vi "initialise.vi"(8 "error in (no error)":errorcluster, 11 "DL090215DataCollection in":refnum<class "DataCollectionMG091001IntrinsicImaging.lvclass">) -> (0 "error out":errorcluster, 3 "DL090215DataCollection out":refnum<class "DataCollectionMG091001IntrinsicImaging.lvclass">)   [LabVIEW 2010, in "DataCollectionMG091001IntrinsicImaging.lvclass"]
uses:
  DataCollectionMG091001IntrinsicImaging.lvclass
  common/enumerations/top-level_component_type_enum.ctl
  DataCollectionDL091104Scaffold/DataCollectionDL091104Scaffold/DataCollectionDL091104Scaffold.lvclass
  common/classes/ImageCollection/ImageCollection/storage_mode_enum.ctl
  DataCollectionMG091001IntrinsicImaging.lvclass/DataCollectionMG091001IntrinsicImaging.ctl
  common/classes/ImageCollection/ImageCollection/ImageCollection.lvclass
  common/classes/ErrorController/ErrorController/class_data.vi
  common/classes/ErrorController/ErrorController/ErrorController.lvclass
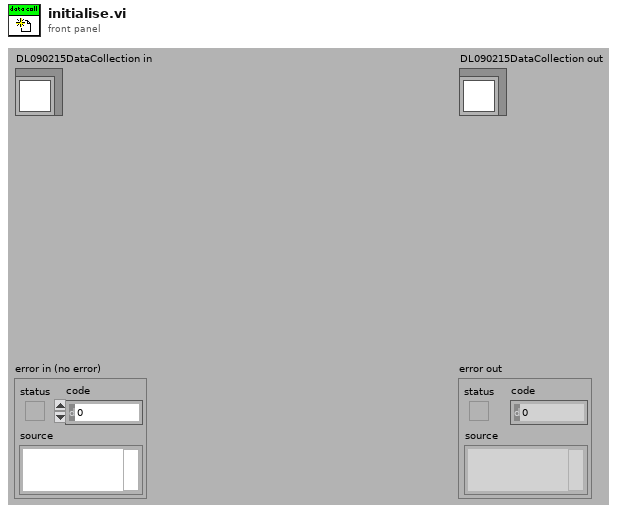
[diagram p1: front panel]
types:
  T1 = typedef "top-level_component_type_enum.ctl" = enum16{"undefined", "ImagingMode", "ScanHead", "DAQ", "ImageAssembler", "Display", "DataCollection", "Analyser", "Stimulator", "ExperimentController", "Instrument", "Stage"}
  T2 = typedef "ImageCollection.lvclass/storage_mode_enum.ctl" = enum16{"RAM", "single files", "multipage TIFF (read-only)"}
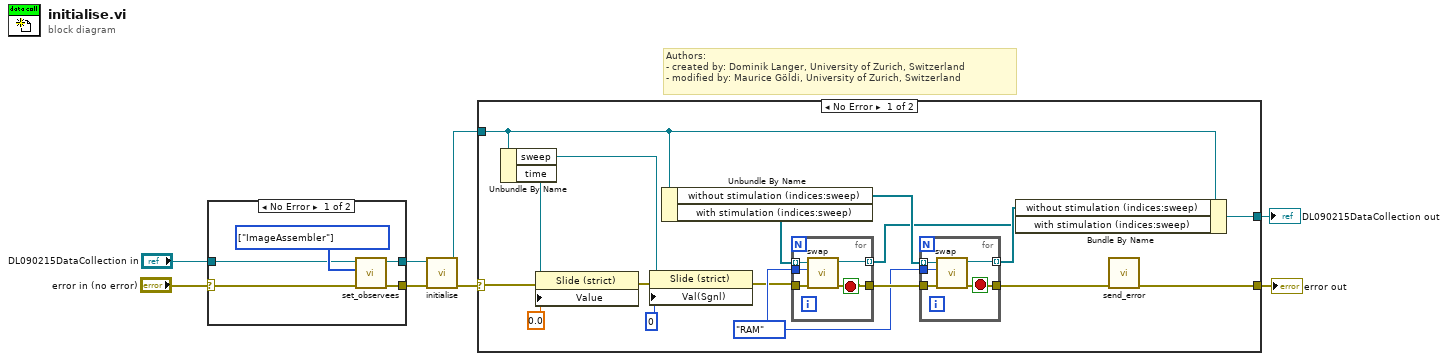
[diagram p0: block diagram]
diagram:
  # "Authors: \n- created by: Dominik Langer, University of Zurich, Switzerland\n- modified by: Maurice Göldi, University of Zurich, Switzerland"
  n1 = case shown="No Error" "error in (no error)" {
    selector: "error in (no error)" -> [w9 w15]
    tunnel: [w12 w15] -> w4
    tunnel: [w11 w14] -> w3
    tunnel: "DL090215DataCollection in" -> [w10 w14]
    frame No Error {
      w13 = T1[] [enum."ImageAssembler"] items=["undefined", "ImagingMode", "ScanHead", "DAQ", "ImageAssembler", "Display", "DataCollection", "Analyser", "Stimulator", "ExperimentController", "Instrument", "Stage"] ("observees")
      n2 = call-dynamic "set_observees.vi"("error in (no error)"=w9, "observees"=w13, "GenericToplevelComponent in"=w10) -> ("error out"=w12:errorcluster, "GenericToplevelComponent out"=w11:refnum<class "DataCollectionMG091001IntrinsicImaging.lvclass">)  [unwired: 7 in]
    }
    frame Error {
    }
  }
  n3 = call-parent "initialise.vi"("error in (no error)"=w4, "DL090215DataCollection in"=w3) -> ("error out"=w8:errorcluster, "DL090215DataCollection out"=w5:refnum<class "DataCollectionMG091001IntrinsicImaging.lvclass">)  [unwired: 8 in]
  n4 = case shown="No Error" w8 {
    selector: w8 -> [w18 w44]
    tunnel: [w27 w43] -> w7
    tunnel: [w16 w44] -> w6
    tunnel: w5 -> [w20 w43]
    frame No Error {
      w26 = storage_mode_enum."RAM" ("target storage mode")
      n5 = Unbundle By Name(w20) -> ("sweep"=w23:refnum<vi>, "time"=w24:refnum<vi>)
      n6 = property class="Slide (strict)"(reference=w24, error in=w18, "Value"=dbl[unit] 0.0) -> (error out=w25:errorcluster)  [unwired: 1 out]
      n7 = property class="Slide (strict)"(reference=w23, error in=w25, "Val(Sgnl)"=0 ("Value (Signaling)")) -> (error out=w19:errorcluster)  [unwired: 1 out]
      n8 = Unbundle By Name(w20) -> ("without stimulation (indices:sweep)"=w30:refnum<class "ImageCollection.lvclass">[], "with stimulation (indices:sweep)"=w32:refnum<class "ImageCollection.lvclass">[])
      n9 = for {
        tunnel: w32 -> [w41] mode=indexing
        tunnel: [w40] -> w28 mode=indexing
        tunnel: w26 -> [w39]
        tunnel: w19 -> [w42]
        tunnel: [w38] -> w31
        stop <- w38 stop-if-true
        n10 = call-dynamic "swap.vi"("error in (no error)"=w42, "target storage mode"=w39, "ImageCollection in"=w41) -> ("error out"=w38:errorcluster, "ImageCollection out"=w40:refnum<class "ImageCollection.lvclass">)  [unwired: 6 in, 1 out]
      }
      n11 = for {
        tunnel: w30 -> [w36] mode=indexing
        tunnel: [w35] -> w29 mode=indexing
        tunnel: w26 -> [w34]
        tunnel: w31 -> [w37]
        tunnel: [w33] -> w17
        stop <- w33 stop-if-true
        n12 = call-dynamic "swap.vi"("error in (no error)"=w37, "target storage mode"=w34, "ImageCollection in"=w36) -> ("error out"=w33:errorcluster, "ImageCollection out"=w35:refnum<class "ImageCollection.lvclass">)  [unwired: 6 in, 1 out]
      }
      n13 = Bundle By Name(cluster=w20, "without stimulation (indices:sweep)"=w29, "with stimulation (indices:sweep)"=w28) -> (w27:refnum<class "DataCollectionMG091001IntrinsicImaging.lvclass">)
      n14 = call "send_error.vi"("error in (no error)"=w17) -> ("error out"=w16:errorcluster)  [unwired: 10 in]
    }
    frame Error {
    }
  }
  "error out" <- w6
  "DL090215DataCollection out" <- w7
